vi "Joules to FE.vi"(5 "J":ext) -> (2 "FE":ext)   [LabVIEW 2021]
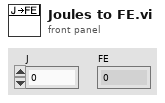
[diagram p1: front panel]
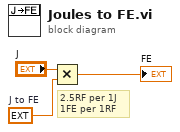
[diagram p0: block diagram]
diagram:
  w3 = ext 0.4  # J to FE
  # "2.5RF per 1J\n1FE per 1RF"
  n1 = Multiply(x="J", y=w3) -> (x*y=→"FE":ext)
